vi "Test.vi"() -> ()   [LabVIEW 2019]
panel:
  in  "Reset Timer":bool
  out "Timer":u32
  in  "Start":bool
  in  "Использовать Алгоритм":bool=TRUE
  in  "Tab Control":T1(tab)
  in  "Порядок действий":T2(array[cluster])=[{"Action"=0, "Val_1"=0.0, "Val_2"=0.0}, {"Action"=1, "Val_1"=30.0, "Val_2"=2500.0}, {"Action"=3, "Val_1"=-10.0, "Val_2"=4000.0}, {"Action"=1, "Val_1"=30.0, "Val_2"=3000.0}, {"Action"=3, "Val_1"=-10.0, "Val_2"=3900.0}, {"Action"=1, "Val_1"=30.0, "Val_2"=6000.0}, {"Action"=3, "Val_1"=10.0, "Val_2"=3800.0}, {"Action"=1, "Val_1"=30.0, "Val_2"=9000.0}, {"Action"=3, "Val_1"=10.0, "Val_2"=3900.0}, {"Action"=6, "Val_1"=0.0, "Val_2"=0.0}] {"Action" items=["Start", "Move_X", "Move_Y", "Rotate_Z", "Gripper_Move", "Stop", "End"]}
  in  "Выбор компоновки":u16(ring)=2 items=["3_Wheels (3 axis)", "3_Wheels (2 axis)", "2_Wheels (2 axis)"]
  in  "Осевое управление":bool=TRUE
  in  "Z_Speed":dbl
  in  "Y_Speed":dbl
  in  "X_Speed":dbl
  out "MotorEnc3":dbl
  in  "MotorSpeed3":dbl
  out "IMU":dbl
  out "US2":dbl
  out "US1":dbl
  out "TitanLimits":bool[](array[boolean])
  out "Analog4":dbl
  out "Analog3":dbl
  out "Analog2":dbl
  out "Analog1":dbl
  in  "MotorSpeed2":dbl
  in  "MotorSpeed1":dbl
  in  "MotorSpeed0":dbl
  out "MotorEnc2":dbl
  out "MotorEnc1":dbl
  out "MotorEnc0":dbl
  in  "Servo_2":dbl(slide) scale=0.0..300.0
  in  "Servo_1":dbl(slide) scale=0.0..300.0
  in  "Stopped LED":bool
  in  "Running LED":bool
  out "Camera":T3(plugin-control)
  out "Вывод ошибок":errorcluster
  in  "stop":bool
  # "Тестовая программа"
  # "Управление"
  # "Моторы"
  # "Датчики"
  # "Камера"
  # "Алгоритмизация"
  # "Подсказка"
  # "В данном разделе задаётся порядок действий которые должен выполнить робот, а так же \"Аргументы\" (X1, X2 и X3 (Возвр.)). Аргументы X1 и X2 - передаются в функцию, а X3 - является возвращемым аргументом.\n   В графе \"Действие\" - выбирается команда которую должен выполнить робот, а в аргументах пишутся значения которые роботу нужно достичь. \n   Описание функций:"
  # "Действие"
  # "X1"
  # "X2"
  # "Описание"
  # "Тестовая программа предназначенна для проверки работы робота и обучения. \nБлок \"Моторы\" - отвечает за контроль вращения скорости моторов и получение данных с инкодеров.\nБлок \"Датчики\" - отвечает за получение данных с аналогвых и цифровых датчиков. \nБлок \"Камера\" - выводит картинку с камеры установленной на роботе.\nИндикатор \"Вывод ошибок\" - выводит сообщения об ошибках в работе программы.\nБлок \"Управление\" - позволяет выбрать компоновку робота используемого для тестирования, а так же управлять им с помощью осевых значений скорости.\nБлок \"Алгоритмизация\" - позволяет на простом примере понять принцип организации выполнения роботом последовательных действий."
  # "Функция \"Start\" - является началом программы и обеспечивает правильное начало её выполнения. Программа не запуститься пока не будет нажата кнопка \"Start\".\n\nВ качестве аргументов:\n \nАргументы не требуются.\n\nX1 - Не используется.\nX2 - Не используется."
  # "Функция \"Move_X - передвигает робота по оси Х (вперёд или назад) с указанной скоростью и указанное время.\n\nВ качестве аргументов:\n \nX1 - Скорость движения (если положительное - движение вперёд, если отрицательное - назад)\nX2 - Время передвижения в мс."
  # "Функция \"Move_Y - передвигает робота по оси Y (вправо или влево) с указанной скоростью и указанное время.\n\nВ качестве аргументов:\n \nX1 - Скорость движения (если положительное - движение вправо, если отрицательное - влево)\nX2 - Время передвижения в мс."
  # "Функция \"Rotate_Z\" - поворачивает робота по часовой или против часовой стрелке.\n\nВ качестве аргументов:\n \nX1 - Скорость поворота (если положиетльное - поворот ПО часовой стрелке, если отрицательное - ПРОТВИ часовой стрелки)\nX2 - Время поворота в мс."
  # "Функция \"Gripper_Move\" - перемещает подъёмный механизм робота в указанное положение.\n\nВ качестве аргументов:\n \nX1 - Позиция подъёмного механизма в диапазоне от 0 до 300.\nX2 - Время перемещения (необходимо указать достаточное для того чтобы подъёмный механизм успел переместиться)."
  # "Функция \"Stop\" - прекращает выполнение действий роботом на поределённое время.\n\nВ качестве аргументов:\n \nX1 - Время ожидания.\nX2 - Не используется."
  # "Функция \"End\" - прекращает выполнение действий роботом и завершает работу программы.\n\nВ качестве аргументов:\n \nАргументов не требуется."
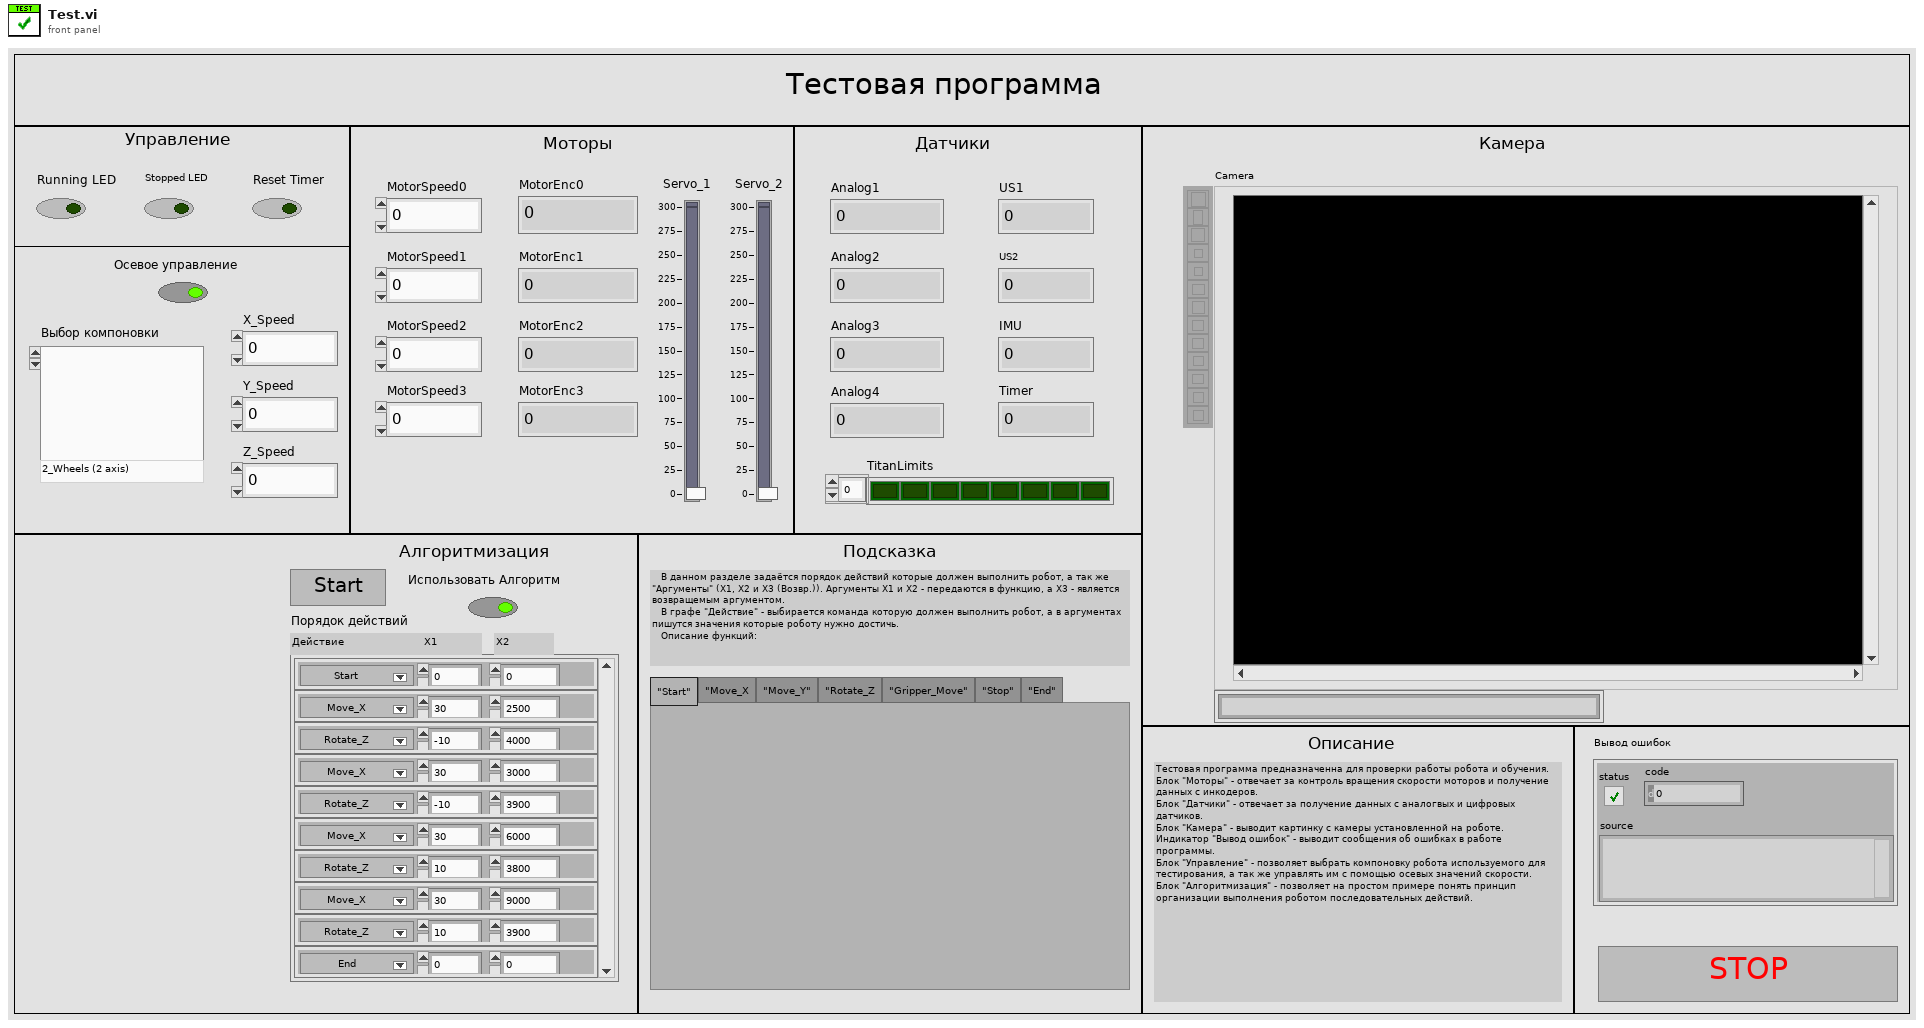
[diagram p1: front panel]
types:
  T1 = enum32{"\"Start\"", "\"Move_X", "\"Move_Y\"", "\"Rotate_Z", "\"Gripper_Move\"", "\"Stop\"", "\"End\""}
  T2 = cluster{"Action":u16, "Val_1":dbl, "Val_2":dbl}[]
  T3 = typedef "IMAQ Image.ctl" = refnum<image>
  T4 = cluster{"CommonLibPath":path, "IsRealRobot":bool, "Talk_data":refnum<k5>, "Listen_data":refnum<k5>, "Camera_data":refnum<k5>, "Camera Image":T3, "Robocad Image":T3}
  T5 = cluster{"MotorSpeed0":dbl, "MotorSpeed1":dbl, "MotorSpeed2":dbl, "MotorSpeed3":dbl, "HCDIO 1":dbl, "HCDIO 2":dbl, "HCDIO 3":dbl, "HCDIO 4":dbl, "HCDIO 5":dbl, "HCDIO 6":dbl, "HCDIO 7":dbl, "HCDIO 8":dbl, "HCDIO 9":dbl, "HCDIO 10":dbl}
  T6 = cluster{"MotorEnc0":dbl, "MotorEnc1":dbl, "MotorEnc2":dbl, "MotorEnc3":dbl, "US1":dbl, "US2":dbl, "Analog1":dbl, "Analog2":dbl, "Analog3":dbl, "Analog4":dbl, "IMU":dbl, "TitanLimits":bool[], "Flexs":bool[], "Camera":T3}
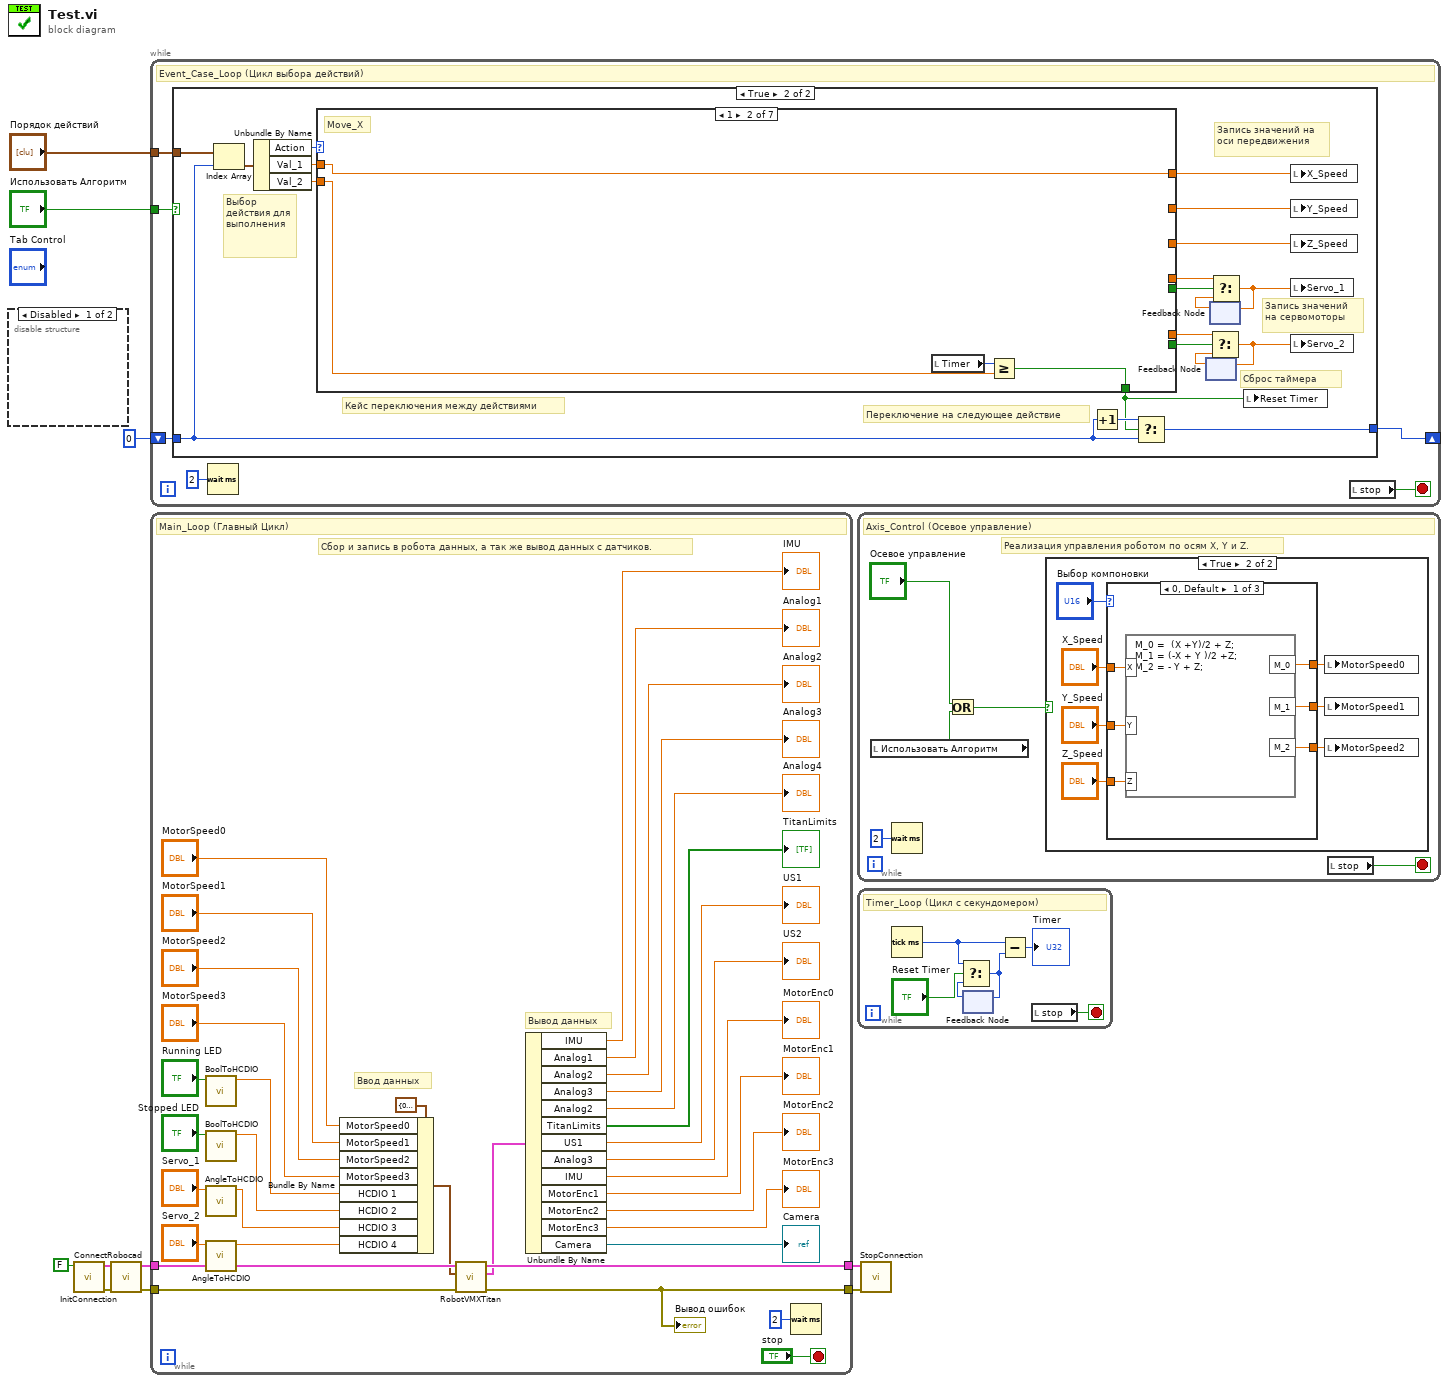
[diagram p0: block diagram]
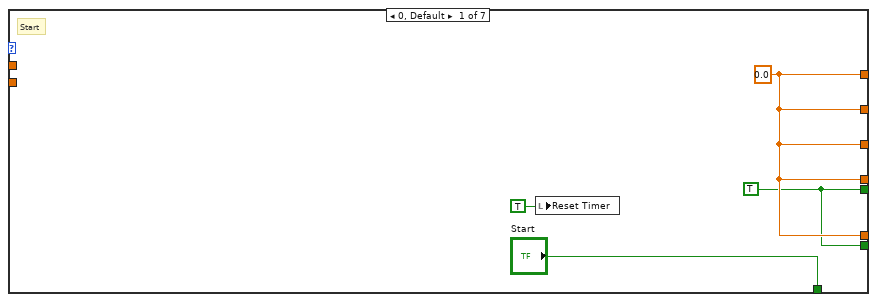
[diagram p3: hidden frame]
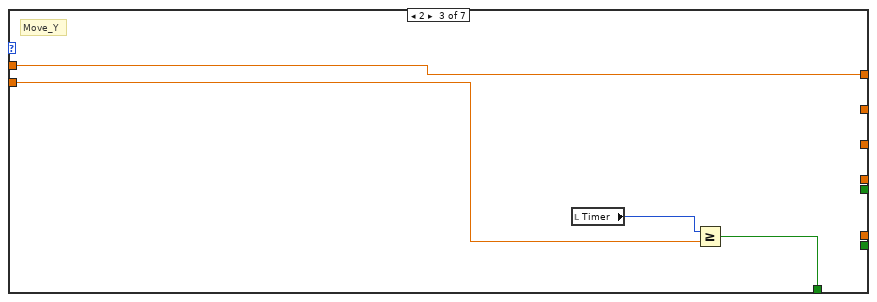
[diagram p4: hidden frame]
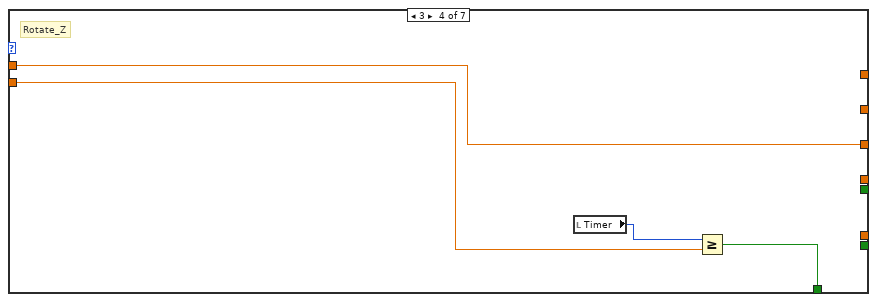
[diagram p5: hidden frame]
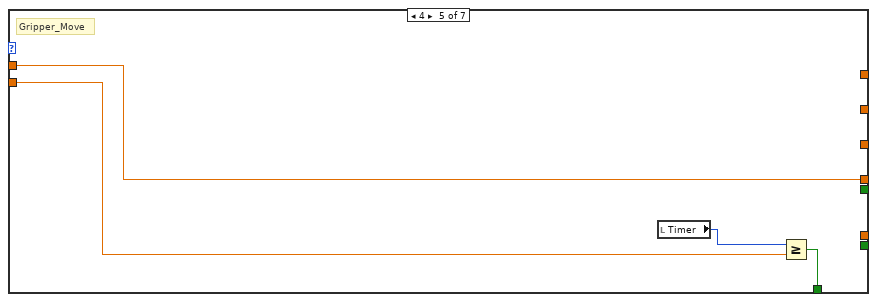
[diagram p6: hidden frame]
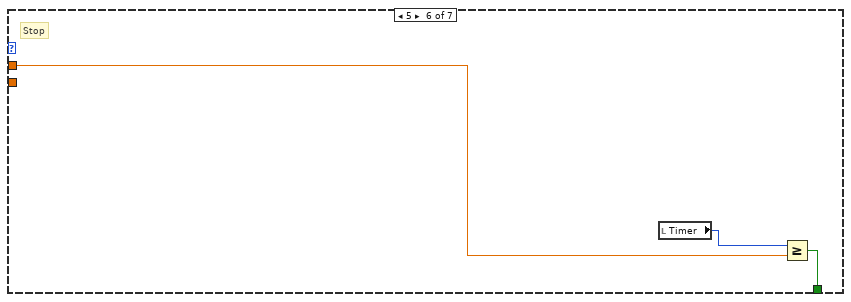
[diagram p7: hidden frame]
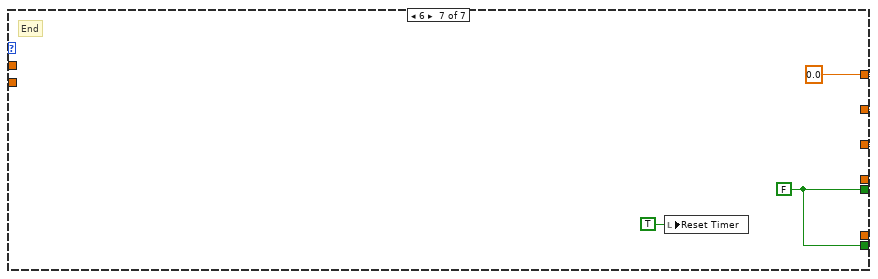
[diagram p8: hidden frame]
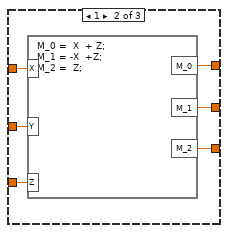
[diagram p11: hidden frame]
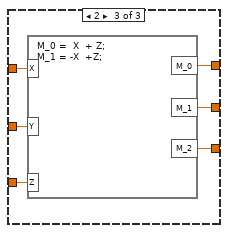
[diagram p12: hidden frame]
diagram:
  n1 = disable-structure shown="Disabled" {
    frame Disabled {
    }
    frame Enabled {
    }
  }
  n2 = call "InitConnection.vi"("IsRealRobot?"=FALSE ("IsRealRobot")) -> ("Error_Out"=w10:errorcluster, "Reference_Out"=w2:T4)  [unwired: 9 in]
  n3 = call "ConnectRobocad.vi"("Error_In"=w10, "Reference_In"=w2) -> ("Error_Out"=w8:errorcluster, "Reference_Out"=w9:T4)  [unwired: 8 in]
  n4 = while {
    shift-right: [w13] -> _
    shift-left: 0 -> [w16]
    tunnel: "Использовать Алгоритм" -> [w15]
    tunnel: "Порядок действий" -> [w14]
    stop <- w12 stop-if-true
    # "Event_Case_Loop (Цикл выбора действий)"
    n5 = case shown="True" w15 {
      tunnel: w16 -> [w17 w35]
      tunnel: w14 -> [_ w36]
      tunnel: [w17 w30] -> w13
      frame False {
      }
      frame True {
        # "Кейс переключения между действиями"
        # "Переключение на следующее действие"
        # "Сброс таймера"
        # "Запись значений на сервомоторы"
        # "Запись значений на оси передвижения"
        # "Выбор действия для выполнения"
        n6 = Index Array(array=w36, index=w35) -> (element=w34:cluster{"Action":u16, "Val_1":dbl, "Val_2":dbl})
        n7 = Unbundle By Name(w34) -> ("Action"=w33:u16, "Val_1"=w32:dbl, "Val_2"=w31:dbl)
        n8 = case shown="1" w33 {
          tunnel: w32 -> [_ w42 w46 w50 w54 w58 _]
          tunnel: w31 -> [_ w44 w47 w51 w55 _ _]
          tunnel: ["Start" w43 w48 w52 w56 w59 _] -> w29
          tunnel: [w40 w42 w46 _ _ _ w63] -> w28
          tunnel: [w40 _ _ _ _ _ _] -> w24
          tunnel: [w40 _ _ _ w54 _ _] -> w25
          tunnel: [w40 _ _ w50 _ _ w63] -> w27
          tunnel: [w40 _ _ _ _ _ w63] -> w26
          tunnel: [w39 _ _ _ _ _ w62] -> w23
          tunnel: [w39 _ _ _ _ _ w62] -> w22
          frame 0, Default {
            w39 = TRUE
            w40 = 0.0
            # "Start"
            n9 = local write "Reset Timer"(TRUE) -> ()
          }
          frame 1 {
            # "Move_X"
            n10 = local read "Timer"() -> (w45:u32)
            n11 = Greater Or Equal?(x=w45, y=w44) -> (x >= y?=w43:bool)
          }
          frame 2 {
            # "Move_Y"
            n12 = local read "Timer"() -> (w49:u32)
            n13 = Greater Or Equal?(x=w49, y=w47) -> (x >= y?=w48:bool)
          }
          frame 3 {
            # "Rotate_Z"
            n14 = local read "Timer"() -> (w53:u32)
            n15 = Greater Or Equal?(x=w53, y=w51) -> (x >= y?=w52:bool)
          }
          frame 4 {
            # "Gripper_Move"
            n16 = local read "Timer"() -> (w57:u32)
            n17 = Greater Or Equal?(x=w57, y=w55) -> (x >= y?=w56:bool)
          }
          frame 5 {
            # "Stop"
            n18 = local read "Timer"() -> (w60:u32)
            n19 = Greater Or Equal?(x=w60, y=w58) -> (x >= y?=w59:bool)
          }
          frame 6 {
            w62 = FALSE
            w63 = 0.0 ("Val_1")
            # "End"
            n20 = local write "Reset Timer"(TRUE ("Reset Timer")) -> ()
          }
        }
        n21 = Increment(x=w35) -> (x+1=w37:i32)
        n22 = Select(t=w37, s=w29, f=w35) -> (s? t:f=w30:i32)
        n23 = feedback #1() -> (w20:dbl)  [unwired: 1 in]
        n24 = feedback #2() -> (w18:dbl)  [unwired: 1 in]
        n25 = Select(t=w24, s=w23, f=w20) -> (s? t:f=w21:dbl)
        n26 = feedback-in #1(w21) -> ()
        n27 = Select(t=w25, s=w22, f=w18) -> (s? t:f=w19:dbl)
        n28 = feedback-in #2(w19) -> ()
        n29 = local write "Reset Timer"(w29) -> ()
        n30 = local write "X_Speed"(w28) -> ()
        n31 = local write "Y_Speed"(w26) -> ()
        n32 = local write "Z_Speed"(w27) -> ()
        n33 = local write "Servo_1"(w19) -> ()
        n34 = local write "Servo_2"(w21) -> ()
      }
    }
    n35 = Wait (ms)(milliseconds to wait=u32 2) -> ()  [unwired: 1 out]
    n36 = local read "stop"() -> (w12:bool)
  }
  n37 = while {
    tunnel: w9 -> [w94]
    tunnel: w8 -> [w96]
    tunnel: [w68] -> w7
    tunnel: [w95] -> w1
    stop <- "stop" stop-if-true
    # "Вывод данных"
    # "Ввод данных"
    # "Сбор и запись в робота данных, а так же вывод данных с датчиков."
    # "Main_Loop (Главный Цикл)"
    n38 = call "BoolToHCDIO.vi"("Bool"="Running LED") -> ("Out"=w90:dbl)  [unwired: 10 in]
    n39 = call "BoolToHCDIO.vi"("Bool"="Stopped LED") -> ("Out"=w87:dbl)  [unwired: 10 in]
    n40 = call "AngleToHCDIO.vi"("Angle"="Servo_1") -> ("Out"=w85:dbl)  [unwired: 10 in]
    n41 = call "AngleToHCDIO.vi"("Angle"="Servo_2") -> ("Out"=w83:dbl)  [unwired: 10 in]
    n42 = Bundle By Name(cluster=T5 {"MotorSpeed0"=0.0, "MotorSpeed1"=0.0, "MotorSpeed2"=0.0, "MotorSpeed3"=0.0, "HCDIO 1"=0.0, "HCDIO 2"=0.0, "HCDIO 3"=0.0, "HCDIO 4"=0.0, "HCDIO 5"=0.0, "HCDIO 6"=0.0, "HCDIO 7"=0.0, "HCDIO 8"=0.0, "HCDIO 9"=0.0, "HCDIO 10"=0.0} ("InCluster"), "MotorSpeed0"="MotorSpeed0", "MotorSpeed1"="MotorSpeed1", "MotorSpeed2"="MotorSpeed2", "MotorSpeed3"="MotorSpeed3", "HCDIO 1"=w90, "HCDIO 2"=w87, "HCDIO 3"=w85, "HCDIO 4"=w83) -> (w66:T5)
    n43 = call "RobotVMXTitan.vi"("Error_In"=w96, "In_Cluster"=w66, "Reference_In"=w94) -> ("Error_Out"=w68:errorcluster, "Out_Cluster"=w67:T6, "Reference_Out"=w95:T4)  [unwired: 6 in]
    "Вывод ошибок" <- w68
    n44 = Unbundle By Name(w67) -> ("IMU"=→"IMU":dbl, "Analog1"=→"Analog1":dbl, "Analog2"=→"Analog2":dbl, "Analog3"=→"Analog3":dbl, "Analog2"=→"Analog4":dbl, "TitanLimits"=→"TitanLimits":bool[], "US1"=→"US1":dbl, "Analog3"=→"US2":dbl, "IMU"=→"MotorEnc0":dbl, "MotorEnc1"=→"MotorEnc1":dbl, "MotorEnc2"=→"MotorEnc2":dbl, "MotorEnc3"=→"MotorEnc3":dbl, "Camera"=→"Camera":T3)
    n45 = Wait (ms)(milliseconds to wait=u32 2) -> ()  [unwired: 1 out]
  }
  n46 = while {
    stop <- w102 stop-if-true
    # "Реализация управления роботом по осям X, Y и Z."
    # "Axis_Control (Осевое управление)"
    n47 = local read "Использовать Алгоритм"() -> (w98:bool)
    n48 = Wait (ms)(milliseconds to wait=u32 2) -> ()  [unwired: 1 out]
    n49 = Or(x="Осевое управление", y=w98) -> (x .or. y?=w100:bool)
    n50 = case shown="True" w100 {
      frame False {
      }
      frame True {
        n51 = case shown="0, Default" "Выбор компоновки" {
          tunnel: "X_Speed" -> [w115 w121 w127]
          tunnel: "Y_Speed" -> [w114 w120 w126]
          tunnel: "Z_Speed" -> [w113 w119 w125]
          tunnel: [w112 w118 w124] -> w106
          tunnel: [w111 w117 w123] -> w105
          tunnel: [w110 w116 w122] -> w104
          frame 0, Default {
            n52 = formula code="M_0 =  (X +Y)/2 + Z;\nM_1 = (-X + Y )/2 +Z;\nM_2 = - Y + Z;"("X"=w115, "Y"=w114, "Z"=w113) -> ("M_0"=w112:dbl, "M_1"=w111:dbl, "M_2"=w110:dbl)
          }
          frame 1 {
            n53 = formula code="M_0 =  X  + Z;\nM_1 = -X  +Z;\nM_2 =  Z;"("X"=w121, "Y"=w120, "Z"=w119) -> ("M_0"=w118:dbl, "M_1"=w117:dbl, "M_2"=w116:dbl)
          }
          frame 2 {
            n54 = formula code="M_0 =  X  + Z;\nM_1 = -X  +Z;"("X"=w127, "Y"=w126, "Z"=w125) -> ("M_0"=w124:dbl, "M_1"=w123:dbl, "M_2"=w122:dbl)
          }
        }
        n55 = local write "MotorSpeed0"(w106) -> ()
        n56 = local write "MotorSpeed1"(w105) -> ()
        n57 = local write "MotorSpeed2"(w104) -> ()
      }
    }
    n58 = local read "stop"() -> (w102:bool)
  }
  n59 = while {
    stop <- w128 stop-if-true
    # "Timer_Loop (Цикл с секундомером)"
    n60 = Tick Count (ms)() -> (millisecond timer value=w133:u32)
    n61 = feedback #3() -> (w132:u32)  [unwired: 1 in]
    n62 = Select(t=w133, s="Reset Timer", f=w132) -> (s? t:f=w131:u32)
    n63 = feedback-in #3(w131) -> ()
    n64 = Subtract(x=w133, y=w131) -> (x-y=→"Timer":u32)
    n65 = local read "stop"() -> (w128:bool)
  }
  n66 = call "StopConnection.vi"("ErrorIn"=w7, "Reference_In"=w1) -> ()  [unwired: 9 in, 1 out]
